vi "Get acceptance limits.vi"(8 "error in (no error)":errorcluster, 10 "section":T1(ring), 11 "configuration file path":path=path "E:/LCU6331 test/Procedure2/Limits_Production.txt") -> (0 "error out":errorcluster, 2 "value":string, 3 "file path":path)   [LabVIEW 2009]
uses:
  <vilib>/Utility/config.llb/Read Key (String).vi
  <vilib>/Utility/config.llb/NI_LVConfig.lvlib
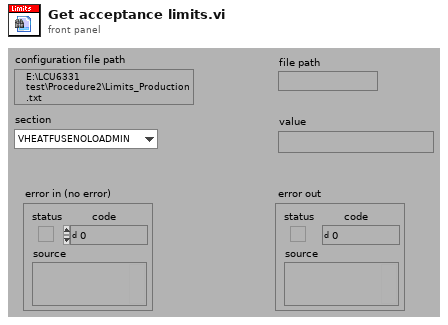
[diagram p1: front panel]
types:
  T1 = enum16{"VHEATFUSENOLOADMIN", "VHEATFUSELOADMAX", "VOVERRIDEDIODEMIN", "TDIFFMAX", "MEASFREQMIN", "MEASFREQMAX", "VMIDDLE", "VUNDER", "VNORESET", "VRESET", "WAITPING", "LRFID", "RFIDUID", "EXTEESIZE", "LCUTYPE", "LCUSUBTYPE", "TEVN", "BOOTVER", "APPVER", "ISLEEPMAX", "TSLEEP", "APPWAIT", "DBWAIT"}
  T2 = typedef "NI_LVConfig.lvlib/Config Data RefNum.ctl" = refnum<k1>
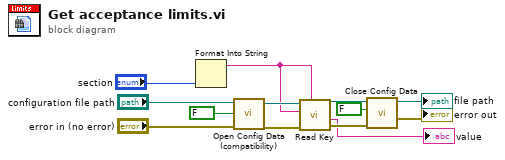
[diagram p0: block diagram]
diagram:
  n1 = Format Into String "Format Into String"("section") -> (resulting string=w2:string)  [unwired: 3 in, 1 out]
  n2 = call <vilib>:"Open Config Data (compatibility).vi"("error in (no error)"="error in (no error)", "create file if necessary (T)"=FALSE ("create file if necessary? (T)"), "configuration file path"="configuration file path") -> ("error out"=w7:errorcluster, "refnum"=w6:T2)  [unwired: 6 in, 1 out]
  n3 = call-poly <vilib>:"Read Key.vi"("section"=w2, "error in (no error)"=w7, "key"=w2, "refnum"=w6) -> ("error out"=w5:errorcluster, "value"=→"value":string, "refnum out"=w4:T2)  [unwired: 2 in, 3 out]
  n4 = call <vilib>:"Close Config Data.vi"("error in (no error)"=w5, "write file if changed (T)"=FALSE ("write configuration file? (T)"), "refnum"=w4) -> ("error out"=→"error out":errorcluster, "file path"=→"file path":path)  [unwired: 7 out]
